vi "MeasureCurrentPos.vi"() -> (1 "Current Position":T1)   [LabVIEW 2011]
uses:
  Main/Motors/MotorPosType.ctl
  Main/Typedefs/XYf.ctl
  PIAxisInfoGlobal.vi
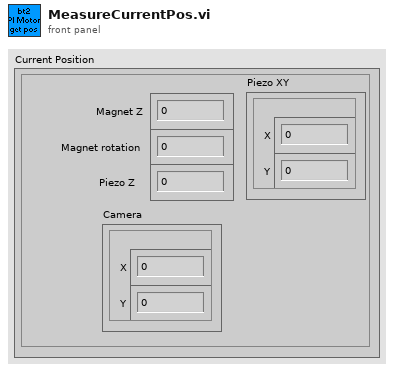
[diagram p1: front panel]
types:
  T1 = typedef "MotorPosType.ctl" = cluster{"Magnet Z":dbl, "Magnet rotation":dbl, "Camera":T2, "Piezo XY":T2, "Piezo Z":dbl}
  T2 = typedef "XYf.ctl" = cluster{"X":sgl, "Y":sgl}
  T3 = typedef "PI_Axis_list.ctl" = cluster{"Piezo X":T4, "Piezo Y":T4, "Piezo Z":T4, "Magnet Z":T4, "Magnet Rotation":T4, "Objective X":T4, "Objective Y":T4}
  T4 = typedef "PI_Axis.ctl" = cluster{"System #":i32, "Axis ID":string, "Multiplier":dbl}
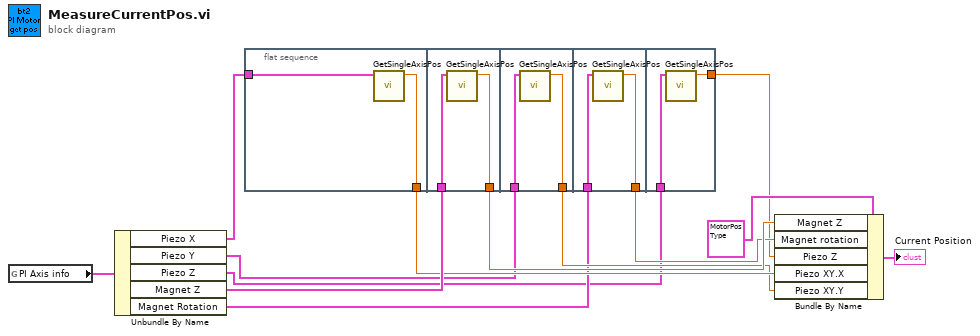
[diagram p0: block diagram]
diagram:
  n1 = global read "PIAxisInfoGlobal.vi" "PI Axis info"() -> (w11:T3)
  n2 = Unbundle By Name(w11) -> ("Piezo X"=w10:T4, "Piezo Y"=w6:T4, "Piezo Z"=w2:T4, "Magnet Z"=w9:T4, "Magnet Rotation"=w4:T4)
  n3 = flat-sequence {
    tunnel: w10 -> [w15]
    tunnel: [w14] -> w8
    tunnel: w9 -> [w17]
    tunnel: [w16] -> w7
    tunnel: w6 -> [w19]
    tunnel: [w18] -> w5
    tunnel: w4 -> [w20]
    tunnel: [w21] -> w3
    tunnel: w2 -> [w23]
    tunnel: [w22] -> w1
    frame #0 {
      n4 = call "GetSingleAxisPos.vi"("Axis"=w15) -> ("Position"=w14:dbl)  [unwired: 9 in, 1 out]
    }
    frame #1 {
      n5 = call "GetSingleAxisPos.vi"("Axis"=w17) -> ("Position"=w16:dbl)  [unwired: 9 in, 1 out]
    }
    frame #2 {
      n6 = call "GetSingleAxisPos.vi"("Axis"=w19) -> ("Position"=w18:dbl)  [unwired: 9 in, 1 out]
    }
    frame #3 {
      n7 = call "GetSingleAxisPos.vi"("Axis"=w20) -> ("Position"=w21:dbl)  [unwired: 9 in, 1 out]
    }
    frame #4 {
      n8 = call "GetSingleAxisPos.vi"("Axis"=w23) -> ("Position"=w22:dbl)  [unwired: 9 in, 1 out]
    }
  }
  n9 = Bundle By Name(cluster=T1 {"Magnet Z"=0.0, "Magnet rotation"=0.0, "Camera"={"X"=0.0, "Y"=0.0}, "Piezo XY"={"X"=0.0, "Y"=0.0}, "Piezo Z"=0.0} ("Current Position"), "Magnet Z"=w7, "Magnet rotation"=w3, "Piezo Z"=w1, "Piezo XY.X"=w8, "Piezo XY.Y"=w5) -> (→"Current Position":T1)
